vi "LS Durability Main (FPGA).vi"() -> ()   [LabVIEW 2013]
uses:
  <vilib>/rvi/Emulation/niFpgaSctlEmulationGetInTimedLoop.vi
  <vilib>/rvi/Emulation/niFpgaEmulationReportErrorSimple.vi
  <vilib>/rvi/Emulation/niFpgaGetClockAttributes.vi
  <vilib>/rvi/DataTransferAndStorage/Container/Common/niFpgaContainerExecOnDevCompGetState.vi
  <vilib>/rvi/FIFO/Fifo_Resource/nirvififoEmulationWriteFpgaImpl.vi
  <vilib>/rvi/DataTransferAndStorage/Container/Common/niFpgaContainerGetUniqueNameForEmu.vi
  <vilib>/rvi/interface/RandomDataEmulation/nirviRandomDataFPGAFIFO.vi
  <vilib>/rvi/interface/RandomDataEmulation/niFpgaRandomDataHandleErrors.vi
  <vilib>/rvi/eio/common/nirviEmuReportErrorAndStop.vi
  <vilib>/rvi/Emulation/niFpgaCriticalErrorInLSC.vi
  <vilib>/rvi/eio/common/nirviEmuTemplateMethod_errors.vi
  <vilib>/rvi/DataTransferAndStorage/Container/XNode/niFpgaContainer.xnode
  <vilib>/rvi/FIFO/Fifo_Resource/niFpgaFifoEmulationRefIn.vi
  <vilib>/eio/EIONode/EIONode.xnode
panel:
  out "FIFO microseconds":u32
  in  "V(T)/R(F)":bool=TRUE
  in  "Resistance In":fxp<+/-,28,17>[](array[numeric])=[0.0, 0.0, 0.0, 0.0, 0.0, 0.0, 0.0, 0.0, 0.0, 0.0, 0.0, 0.0]
  in  "Subtract Noise":bool
  out "Anomaly Array":fxp<+/-,29,18>[](array[numeric])
  in  "Enable2ndStepCheck":bool
  out "Anomaly Resamples":fxp<+/-,28,17>[](array[numeric])
  in  "Anomaly Threshold":fxp<+/-,28,17>=0.02978515625
  out "Bank2Active":bool
  out "Bank1Active":bool
  out "Bank2On":bool
  out "Bank1On":bool
  in  "Enable Readings":bool[](array[boolean])=[FALSE, FALSE, FALSE, FALSE, FALSE, FALSE, FALSE, FALSE, FALSE, FALSE, FALSE, FALSE]
  in  "Opens Resets":bool[](array[boolean])=[FALSE, FALSE, FALSE, FALSE, FALSE, FALSE, FALSE, FALSE, FALSE, FALSE, FALSE, FALSE]
  in  "Enable Opens":bool[](array[boolean])=[FALSE, FALSE, FALSE, FALSE, FALSE, FALSE, FALSE, FALSE, FALSE, FALSE, FALSE, FALSE]
  out "Opens Detected":u16[](array[numeric])
  out "Opens Loop Time (usec)":u32=1000
  in  "Bank2(Pulse/Const)":bool
  in  "Bank2Const(On/Off)":bool
  out "Anomalies (Last Cycle)":i32[](array[numeric])
  out "Cycle Starts":bool[](array[boolean])
  out "Anomalies (Total)":i32[](array[numeric])
  out "Anomalies/Cycle":i32[](array[numeric])
  in  "Normal Steps":u32=98
  out "Cycles":u32[](array[numeric])
  out "Anomaly Loop Time (usec)":u32=1000
  out "Steps":u32[](array[numeric])
  in  "Step Threshold":fxp<+/-,28,17>=0.02978515625
  in  "Enable Anomalies":bool[](array[boolean])=[FALSE, FALSE, FALSE, FALSE, FALSE, FALSE, FALSE, FALSE, FALSE, FALSE, FALSE, FALSE]
  in  "Anomaly Resets":bool[](array[boolean])=[FALSE, FALSE, FALSE, FALSE, FALSE, FALSE, FALSE, FALSE, FALSE, FALSE, FALSE, FALSE]
  in  "Bank1Const(On/Off)":bool
  in  "Bank1(Pulse/Const)":bool
  in  "PWM Period (Ticks)":u32=4000000
  in  "Duty (Ticks)":i32=2000000
  in  "Invert PWM?":bool=TRUE
  in  "Cycle Resets":bool[](array[boolean])=[FALSE, FALSE, FALSE, FALSE, FALSE, FALSE, FALSE, FALSE, FALSE, FALSE, FALSE, FALSE]
  in  "Points to Avg":i32=20
  in  "Enable Cycles":bool[](array[boolean])=[FALSE, FALSE, FALSE, FALSE, FALSE, FALSE, FALSE, FALSE, FALSE, FALSE, FALSE, FALSE]
  out "Total Cycles":u32[](array[numeric])
  in  "Cycle Threshold":fxp<+/-,28,17>=1.2001953125
  out "AI Avg Loop Time (usec)":u32=1000
  out "Analog Inputs":fxp<+/-,28,17>[](array[numeric])
  out "AI Loop Time (usec)":u32=70
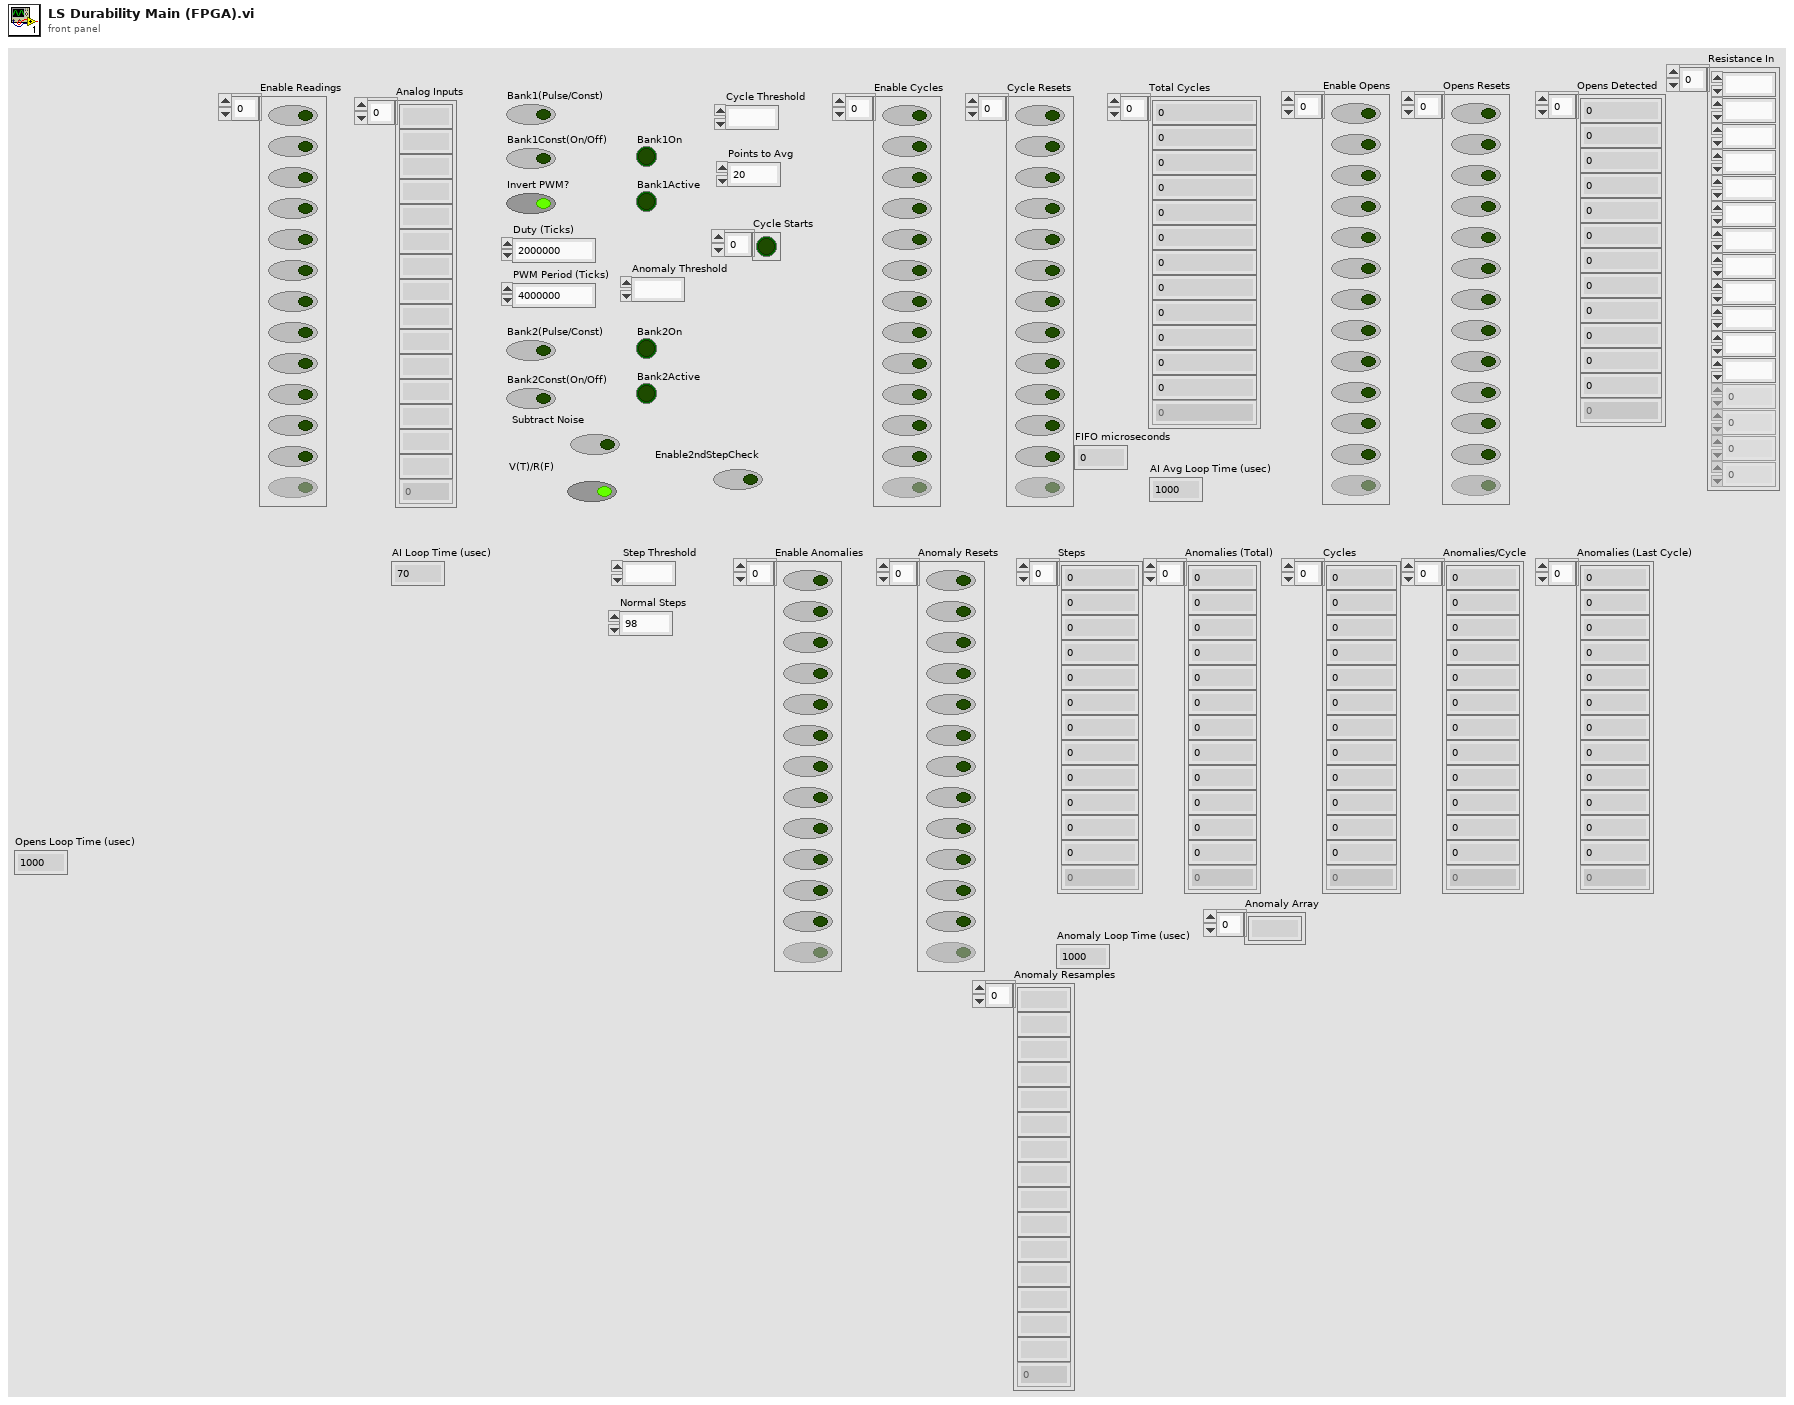
[diagram p1: front panel]
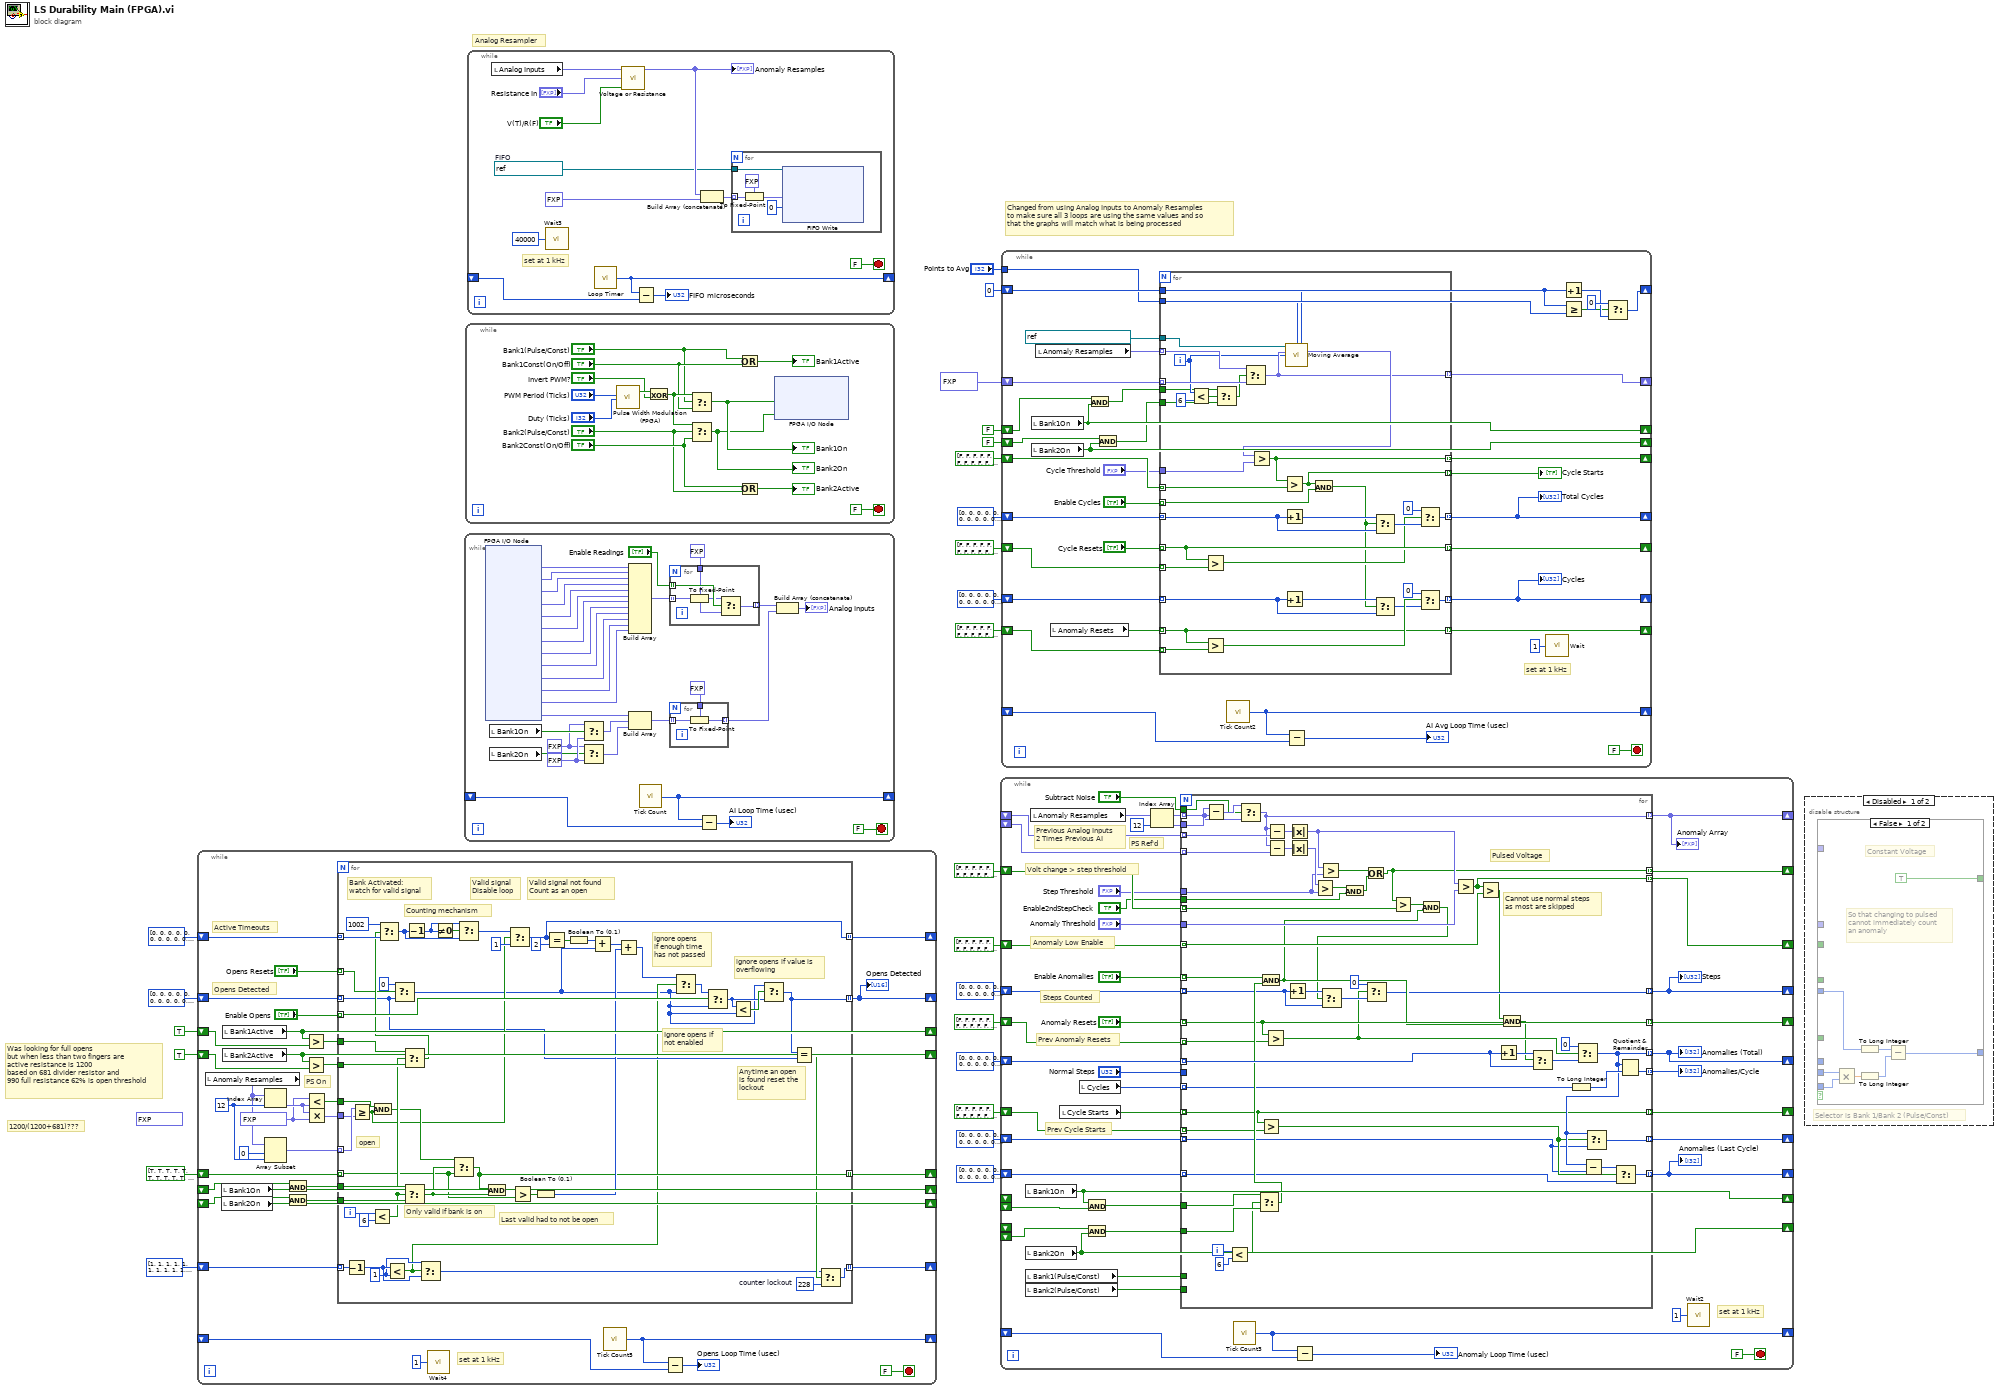
[diagram p0: block diagram]
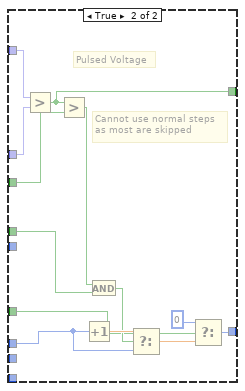
[diagram p2: hidden frame]
diagram:
  (unwired) fxp<+,8,0> 0.94921875
  # "Changed from using Analog Inputs to Anomaly Resamples\nto make sure all 3 loops are using the same values and so\nthat the graphs will match what is being processed"
  # "Analog Resampler"
  # "1200/(1200+681)???"
  # "Was looking for full opens\nbut when less than two fingers are\nactive resistance is 1200\nbased on 681 divider resistor and\n990 full resistance 62% is open threshold"
  n1 = while {
    shift-right: [w57] -> _
    shift-left: _ -> [w56]
    shift-right: [w28] -> _
    shift-left: u8[] [0, 0, 0, 0, 0, 0, 0, 0, 0, 0, 0, 0] -> [w52]
    shift-right: [w37] -> _
    shift-left: u16[] [0, 0, 0, 0, 0, 0, 0, 0, 0, 0, 0, 0] -> [w38]
    shift-right: [w44] -> _
    shift-left: bool[] [TRUE, TRUE, TRUE, TRUE, TRUE, TRUE, TRUE, TRUE, TRUE, TRUE, TRUE, TRUE] -> [w43]
    shift-right: [w42] -> _
    shift-left: TRUE ("Bank2Active") -> [w40]
    shift-right: [w41] -> _
    shift-left: TRUE ("Bank1Active") -> [w39]
    shift-right: [w31] -> _
    shift-left: _ -> [w29]
    shift-right: [w32] -> _
    shift-left: _ -> [w30]
    shift-right: [w26] -> _
    shift-left: u16[] [1, 1, 1, 1, 1, 1, 1, 1, 1, 1, 1, 1] -> [w27]
    stop <- FALSE stop-if-true
    w45 = fxp<+,8,0> 0.62109375
    w54 = 12 ("length")
    # "Opens Detected"
    # "Active Timeouts"
    # "PS On"
    # "set at 1 kHz"
    n2 = local read "Anomaly Resamples"() -> (w25:fxp<+/-,28,17>[])
    n3 = local read "Bank1On"() -> (w32:bool)
    n4 = local read "Bank2On"() -> (w31:bool)
    n5 = local read "Bank1Active"() -> (w41:bool)
    n6 = local read "Bank2Active"() -> (w42:bool)
    n7 = Index Array(array=w25, index=w54) -> (element=w46:fxp<+/-,28,17>)
    n8 = Array Subset(array=w25, index=0, length=w54) -> (w47:fxp<+/-,28,17>[])
    n9 = And(x=w30, y=w32) -> (x .and. y?=w34:bool)
    n10 = And(x=w29, y=w31) -> (x .and. y?=w33:bool)
    n11 = Greater?(x=w41, y=w39) -> (0:w51:bool)
    n12 = Greater?(x=w42, y=w40) -> (0:w50:bool)
    n13 = Less?(x=w45, y=w46) -> (x < y?=w49:bool)
    n14 = Multiply(x=w46, y=w45) -> (x*y=w48:fxp<+/-,36,17>)
    n15 = for {
      tunnel: w34 -> [w106]
      tunnel: w33 -> [w105]
      tunnel: w51 -> [w103]
      tunnel: w50 -> [w104]
      tunnel: w52 -> [w64] mode=indexing
      tunnel: w38 -> [w91] mode=indexing
      tunnel: "Opens Resets" -> [w75] mode=indexing
      tunnel: "Enable Opens" -> [w89] mode=indexing
      tunnel: [w65] -> w28 mode=indexing
      tunnel: w48 -> [w86]
      tunnel: w47 -> [w87] mode=indexing
      tunnel: w49 -> [w85]
      tunnel: [w76] -> w44 mode=indexing
      tunnel: w43 -> [w81] mode=indexing
      tunnel: [w79] -> w37 mode=indexing
      tunnel: w27 -> [w70] mode=indexing
      tunnel: [w66] -> w26 mode=indexing
      i -> [w108]
      w67 = u16 228  # counter lockout
      w71 = u16 1 ("y")
      # "Ignore opens if\nnot enabled"
      # "Ignore opens\nif enough time\nhas not passed"
      # "Anytime an open\nis found reset the\nlockout"
      # "ignore opens if value is\noverflowing"
      # "Last valid had to not be open"
      # "Only valid if bank is on"
      # "open"
      # "Valid signal not found\nCount as an open"
      # "Valid signal\nDisable loop"
      # "Counting mechanism"
      # "Bank Activated:\nwatch for valid signal"
      n16 = Decrement(x=w70) -> (x-1=w72:u16)
      n17 = Greater Or Equal?(x=w87, y=w86) -> (x >= y?=w78:bool)
      n18 = Less?(x=w108, y=6) -> (x < y?=w102:bool)
      n19 = And(x=w85, y=w78) -> (x .and. y?=w84:bool)
      n20 = Less?(x=w72, y=w71) -> (x < y?=w61:bool)
      n21 = Select(t=u16 0, s=w75, f=w64) -> (s? t:f=w60:u16)
      n22 = Select(t=w103, s=w102, f=w104) -> (s? t:f=w88:bool)
      n23 = Select(t=u16 1002, s=w88, f=w91) -> (s? t:f=w90:u16)
      n24 = Select(t=w106, s=w102, f=w105) -> (s? t:f=w83:bool)
      n25 = Decrement(x=w90) -> (x-1=w95:u16)
      n26 = Select(t=w71, s=w61, f=w72) -> (s? t:f=w68:u16)
      n27 = Not Equal To 0?(x=w95) -> (x != 0?=w94:bool)
      n28 = Select(t=w84, s=w83, f=w81) -> (s? t:f=w76:bool)
      n29 = Select(t=w95, s=w94, f=w90) -> (s? t:f=w96:u16)
      n30 = And(x=w76, y=w83) -> (x .and. y?=w77:bool)
      n31 = Select(t=w96, s=w78, f=u16 1) -> (s? t:f=w79:u16)
      n32 = Greater?(x=w77, y=w81) -> (0:w82:bool)
      n33 = Boolean To (0,1)(Boolean=w82) -> (0, 1=w80:i16)
      n34 = Equal?(x=w79, y=u16 2) -> (x = y?=w98:bool)
      n35 = Boolean To (0,1)(Boolean=w98) -> (0, 1=w99:i16)
      n36 = Add(x=w99, y=w60) -> (x+y=w100:u16)
      n37 = Add(x=w100, y=w80) -> (x+y=w62:u16)
      n38 = Select(t=w62, s=w61, f=w60) -> (s? t:f=w63:u16)
      n39 = Select(t=w63, s=w89, f=w60) -> (s? t:f=w73:u16)
      n40 = Less?(x=w73, y=w60) -> (x < y?=w74:bool)
      n41 = Select(t=w60, s=w74, f=w73) -> (s? t:f=w65:u16)
      n42 = Equal?(x=w65, y=w64) -> (x = y?=w69:bool)
      n43 = Select(t=w68, s=w69, f=w67) -> (s? t:f=w66:u16)
    }
    "Opens Detected" <- w28
    n44 = call "Wait4"("Count(mSec)"=u32 1) -> ()  [unwired: 1 out]
    n45 = call "Tick Count5"() -> ("Tick Count(uSec)"=w57:u32)
    n46 = Subtract(x=w57, y=w56) -> (x-y=→"Opens Loop Time (usec)":u32)
  }
  n47 = while {
    shift-right: [w138] -> _
    shift-left: _ -> [w137]
    stop <- FALSE stop-if-true
    w111 = fxp<+/-,24,5> 1.0 ("AI13")
    w114 = fxp<+/-,24,5> 0.0 ("AI13")
    n48 = xnode "FPGA I/O Node"() -> ("AI0"=w135:fxp<+/-,24,5>, "AI1"=w134:fxp<+/-,24,5>, "AI2"=w133:fxp<+/-,24,5>, "AI3"=w132:fxp<+/-,24,5>, "AI4"=w131:fxp<+/-,24,5>, "AI5"=w130:fxp<+/-,24,5>, "AI6"=w129:fxp<+/-,24,5>, "AI7"=w128:fxp<+/-,24,5>, "AI8"=w127:fxp<+/-,24,5>, "AI9"=w126:fxp<+/-,24,5>, "AI10"=w125:fxp<+/-,24,5>, "AI11"=w124:fxp<+/-,24,5>, "AI12"=w121:fxp<+/-,24,5>)  [unwired: 13 in, 13 out]
    n49 = local read "Bank1On"() -> (w113:bool)
    n50 = local read "Bank2On"() -> (w112:bool)
    n51 = Select(t=w111, s=w113, f=w114) -> (s? t:f=w110:fxp<+/-,24,5>)
    n52 = Select(t=w111, s=w112, f=w114) -> (s? t:f=w109:fxp<+/-,24,5>)
    n53 = Build Array(w135, w134, w133, w132, w131, w130, w129, w128, w127, w126, w125, w124) -> (w123:fxp<+/-,24,5>[])
    n54 = Build Array(w121, w110, w109) -> (w119:fxp<+/-,24,5>[])
    n55 = call "Tick Count"() -> ("Tick Count(uSec)"=w138:u32)
    n56 = for {
      tunnel: w123 -> [w147] mode=indexing
      tunnel: fxp<+/-,28,17> 0.0 ("AI0") -> [w144]
      tunnel: [w143] -> w117 mode=indexing
      tunnel: "Enable Readings" -> [w146] mode=indexing
      n57 = To Fixed-Point(fixed-point type=w144, number=w147) -> (fixed-point=w145:fxp<+/-,28,17>)
      n58 = Select(t=w145, s=w146, f=w144) -> (s? t:f=w143:fxp<+/-,28,17>)
    }
    n59 = for {
      tunnel: w119 -> [w142] mode=indexing
      tunnel: fxp<+/-,28,17> 0.0 ("AI0") -> [w141]
      tunnel: [w140] -> w118 mode=indexing
      n60 = To Fixed-Point(fixed-point type=w141, number=w142) -> (fixed-point=w140:fxp<+/-,28,17>)
    }
    n61 = Subtract(x=w138, y=w137) -> (x-y=→"AI Loop Time (usec)":u32)
    n62 = Build Array (concatenate)(w117, w118) -> (→"Analog Inputs":fxp<+/-,28,17>[])
  }
  n63 = while {
    stop <- FALSE stop-if-true
    n64 = call "Pulse Width Modulation (FPGA).vi"("PWM Period (Ticks)"="PWM Period (Ticks)", "PWM Duty Cycle (Ticks)"="Duty (Ticks)") -> ("PWM DO"=w158:bool)  [unwired: 14 in, 3 out]
    n65 = Exclusive Or(1:"Invert PWM?", 2:w158) -> (0:w156:bool)
    n66 = Select(t=w156, s="Bank1(Pulse/Const)", f="Bank1Const(On/Off)") -> (s? t:f=w155:bool)
    "Bank1On" <- w155
    n67 = Select(t=w156, s="Bank2(Pulse/Const)", f="Bank2Const(On/Off)") -> (s? t:f=w154:bool)
    "Bank2On" <- w154
    n68 = Or(x="Bank1(Pulse/Const)", y="Bank1Const(On/Off)") -> (x .or. y?=→"Bank1Active":bool)
    n69 = Or(x="Bank2Const(On/Off)", y="Bank2(Pulse/Const)") -> (x .or. y?=→"Bank2Active":bool)
    n70 = xnode "FPGA I/O Node"("RMC/DIO0"=w155, "RMC/DIO1"=w154) -> ()  [unwired: 3 in, 3 out]
  }
  n71 = while {
    shift-right: [w163] -> _
    shift-left: _ -> [w164]
    stop <- FALSE stop-if-true
    w165 = refnum<k21> "Analog Data"  # FIFO
    # "set at 1 kHz"
    n72 = local read "Analog Inputs"() -> (w169:fxp<+/-,28,17>[])
    n73 = call "Wait3"("Count(Ticks)"=u32 40000 ("Count(mSec)")) -> ()  [unwired: 1 out]
    n74 = call "Loop Timer"() -> ("Tick Count(uSec)"=w163:u32)  [unwired: 1 in]
    n75 = call "Voltage or Resistance.vi"("Data In"=w169, "Resistance In"="Resistance In", "V(T)/R(F)"="V(T)/R(F)") -> ("Data Out"=w168:fxp<+/-,28,17>[])  [unwired: 12 in]
    "Anomaly Resamples" <- w168
    n76 = Subtract(x=w163, y=w164) -> (x-y=→"FIFO microseconds":u32)
    n77 = Build Array (concatenate)(w168, fxp<+/-,28,17> -15.0 ("AI0")) -> (w172:fxp<+/-,28,17>[])
    n78 = for {
      tunnel: w165 -> [w178]
      tunnel: w172 -> [w177] mode=indexing
      n79 = To Fixed-Point(fixed-point type=fxp<+/-,18,11> 0.0 ("AI0"), number=w177) -> (fixed-point=w176:fxp<+/-,18,11>)
      n80 = xnode "FIFO Write"("Element"=w176, "Timeout"=0, "FIFO In"=w178) -> ()  [unwired: 2 out]
    }
  }
  n81 = while {
    shift-right: [w220] -> _
    shift-left: _ -> [w219]
    shift-right: [w212] -> _
    shift-left: bool[] [FALSE, FALSE, FALSE, FALSE, FALSE, FALSE, FALSE, FALSE, FALSE, FALSE, FALSE, FALSE] -> [w211]
    shift-right: [w209] -> _
    shift-left: u32[] [0, 0, 0, 0, 0, 0, 0, 0, 0, 0, 0, 0] -> [w208]
    shift-right: [w207] -> _
    shift-left: bool[] [FALSE, FALSE, FALSE, FALSE, FALSE, FALSE, FALSE, FALSE, FALSE, FALSE, FALSE, FALSE] -> [w204]
    shift-right: [w214] -> _
    shift-left: _ -> [w213]
    shift-right: [w201] -> _
    shift-left: bool[] [FALSE, FALSE, FALSE, FALSE, FALSE, FALSE, FALSE, FALSE, FALSE, FALSE, FALSE, FALSE] -> [w200]
    shift-right: [w199] -> _
    shift-left: i32[] [0, 0, 0, 0, 0, 0, 0, 0, 0, 0, 0, 0] -> [w197]
    shift-right: [w198] -> _
    shift-left: i32[] [0, 0, 0, 0, 0, 0, 0, 0, 0, 0, 0, 0] -> [w196]
    shift-right: [w188] -> _
    shift-left: _ -> [_]
    shift-right: [w215] -> _
    shift-left: _ -> [_]
    shift-right: [w193] -> _
    shift-left: i32[] [0, 0, 0, 0, 0, 0, 0, 0, 0, 0, 0, 0] -> [w192]
    shift-right: [w189] -> _
    shift-left: bool[] [FALSE, FALSE, FALSE, FALSE, FALSE, FALSE, FALSE, FALSE, FALSE, FALSE, FALSE, FALSE] -> [w190]
    shift-left: _ -> [w186]
    shift-left: _ -> [w187]
    shift-left: _ -> [w184]
    stop <- FALSE stop-if-true
    # "PS Ref'd"
    # "Anomaly Low Enable"
    # "Prev Cycle Starts"
    # "Prev Anomaly Resets"
    # "Steps Counted"
    # "Volt change > step threshold"
    # "Previous Analog Inputs\n2 Times Previous AI"
    # "set at 1 kHz"
    n82 = local read "Bank1On"() -> (w188:bool)
    n83 = local read "Bank2On"() -> (w215:bool)
    n84 = local read "Bank1(Pulse/Const)"() -> (w195:bool)
    n85 = local read "Bank2(Pulse/Const)"() -> (w194:bool)
    n86 = local read "Anomaly Resamples"() -> (w182:fxp<+/-,28,17>[])
    n87 = local read "Cycle Starts"() -> (w202:bool[])
    n88 = local read "Cycles"() -> (w203:u32[])
    n89 = And(x=w188, y=w187) -> (x .and. y?=w217:bool)
    n90 = And(x=w186, y=w215) -> (x .and. y?=w216:bool)
    n91 = Index Array(array=w182, index=12) -> (element=w181:fxp<+/-,28,17>)
    n92 = for {
      tunnel: w182 -> [w225] mode=indexing
      tunnel: [w232] -> w212 mode=indexing
      tunnel: w211 -> [w253] mode=indexing
      tunnel: w208 -> [w246] mode=indexing
      tunnel: [w245] -> w209 mode=indexing
      tunnel: "Step Threshold" -> [w234]
      tunnel: "Enable Anomalies" -> [w272] mode=indexing
      tunnel: "Anomaly Resets" -> [w255] mode=indexing
      tunnel: [w255] -> w207 mode=indexing
      tunnel: w204 -> [w256] mode=indexing
      tunnel: [w226] -> w214 mode=indexing
      tunnel: w213 -> [w273] mode=indexing
      tunnel: "Normal Steps" -> [_]
      tunnel: w203 -> [w263] mode=indexing
      tunnel: [w262] -> w205 mode=indexing
      tunnel: [w264] -> w193 mode=indexing
      tunnel: w202 -> [w258] mode=indexing
      tunnel: [w258] -> w201 mode=indexing
      tunnel: w200 -> [w259] mode=indexing
      tunnel: [w261] -> w199 mode=indexing
      tunnel: w197 -> [w244] mode=indexing
      tunnel: [w260] -> w198 mode=indexing
      tunnel: w196 -> [w243] mode=indexing
      tunnel: w217 -> [w280]
      tunnel: w216 -> [w279]
      tunnel: w195 -> [_]
      tunnel: w194 -> [_]
      tunnel: w192 -> [w275] mode=indexing
      tunnel: "Anomaly Threshold" -> [w269]
      tunnel: w190 -> [w268] mode=indexing
      tunnel: [w267] -> w189 mode=indexing
      tunnel: w184 -> [w236] mode=indexing
      tunnel: "Enable2ndStepCheck" -> [w229]
      tunnel: w181 -> [w228]
      tunnel: "Subtract Noise" -> [w224]
      i -> [w278]
      # "Cannot use normal steps\nas most are skipped"
      # "Pulsed Voltage"
      n93 = Subtract(x=w228, y=w225) -> (x-y=w227:fxp<+/-,29,18>)
      n94 = Less?(x=w278, y=6) -> (x < y?=w276:bool)
      n95 = Select(t=w227, s=w224, f=w225) -> (s? t:f=w226:fxp<+/-,29,18>)
      n96 = Select(t=w280, s=w276, f=w279) -> (s? t:f=w271:bool)
      n97 = And(x=w272, y=w271) -> (x .and. y?=w252:bool)
      n98 = Greater?(x=w258, y=w259) -> (0:w257:bool)
      n99 = Greater?(x=w255, y=w256) -> (0:w248:bool)
      n100 = Subtract(x=w226, y=w273) -> (x-y=w274:fxp<+/-,30,19>)
      n101 = Subtract(x=w226, y=w236) -> (x-y=w237:fxp<+/-,30,19>)
      n102 = Increment(x=w246) -> (x+1=w249:u32)
      n103 = Absolute Value(x=w274) -> (abs(x)=w270:fxp<+,29,18>)
      n104 = Absolute Value(x=w237) -> (abs(x)=w235:fxp<+,29,18>)
      n105 = Greater?(x=w235, y=w234) -> (0:w231:bool)
      n106 = Greater?(x=w270, y=w234) -> (0:w233:bool)
      n107 = And(x=w231, y=w229) -> (x .and. y?=w230:bool)
      n108 = Or(x=w233, y=w230) -> (x .or. y?=w232:bool)
      n109 = Greater?(x=w232, y=w253) -> (0:w254:bool)
      n110 = And(x=w254, y=w252) -> (x .and. y?=w247:bool)
      n111 = Select(t=w249, s=w247, f=w246) -> (s? t:f=w250:u32)
      n112 = Select(t=u32 0, s=w248, f=w250) -> (s? t:f=w245:u32)
      n113 = Greater?(x=w270, y=w269) -> (0:w267:bool)
      n114 = Greater?(x=w267, y=w268) -> (0:w238:bool)
      n115 = Increment(x=w275) -> (x+1=w240:i32)
      n116 = And(x=w238, y=w252) -> (x .and. y?=w239:bool)
      n117 = Select(t=w240, s=w239, f=w275) -> (s? t:f=w241:i32)
      n118 = To Long Integer(number=w263) -> (32bit integer=w265:i32)
      n119 = Select(t=0, s=w248, f=w241) -> (s? t:f=w264:i32)
      n120 = Subtract(x=w264, y=w244) -> (x-y=w266:i32)
      n121 = Select(t=w264, s=w257, f=w244) -> (s? t:f=w261:i32)
      n122 = Select(t=w266, s=w257, f=w243) -> (s? t:f=w260:i32)
      n123 = Quotient & Remainder(x=w264, y=w265) -> (floor(x/y)=w262:i32)  [unwired: 1 out]
    }
    "Steps" <- w209
    "Anomalies/Cycle" <- w205
    "Anomalies (Total)" <- w193
    "Anomalies (Last Cycle)" <- w198
    "Anomaly Array" <- w214
    n124 = call "Tick Count3"() -> ("Tick Count(uSec)"=w220:u32)
    n125 = Subtract(x=w220, y=w219) -> (x-y=→"Anomaly Loop Time (usec)":u32)
    n126 = call "Wait2"("Count(mSec)"=u32 1) -> ()  [unwired: 1 out]
  }
  n127 = while {
    shift-right: [w310] -> _
    shift-left: 0 ("Moving Point Index") -> [w311]
    shift-right: [w307] -> _
    shift-left: _ -> [w306]
    shift-right: [w305] -> _
    shift-left: bool[] [FALSE, FALSE, FALSE, FALSE, FALSE, FALSE, FALSE, FALSE, FALSE, FALSE, FALSE, FALSE] -> [w304]
    shift-right: [w302] -> _
    shift-left: u32[] [0, 0, 0, 0, 0, 0, 0, 0, 0, 0, 0, 0] -> [w303]
    tunnel: "Points to Avg" -> [w299]
    shift-right: [w297] -> _
    shift-left: bool[] [FALSE, FALSE, FALSE, FALSE, FALSE, FALSE, FALSE, FALSE, FALSE, FALSE, FALSE, FALSE] -> [w296]
    shift-right: [w291] -> _
    shift-left: u32[] [0, 0, 0, 0, 0, 0, 0, 0, 0, 0, 0, 0] -> [w293]
    shift-right: [w294] -> _
    shift-left: bool[] [FALSE, FALSE, FALSE, FALSE, FALSE, FALSE, FALSE, FALSE, FALSE, FALSE, FALSE, FALSE] -> [w295]
    shift-right: [w287] -> _
    shift-left: FALSE -> [w285]
    shift-right: [w283] -> _
    shift-left: FALSE -> [w284]
    shift-right: [w288] -> _
    shift-left: fxp<+/-,28,17>[] [0.0, 0.0, 0.0, 0.0, 0.0, 0.0, 0.0, 0.0, 0.0, 0.0, 0.0, 0.0] ("Analog Inputs") -> [w289]
    stop <- FALSE stop-if-true
    # "set at 1 kHz"
    n128 = local read "Bank1On"() -> (w287:bool)
    n129 = local read "Bank2On"() -> (w283:bool)
    n130 = local read "Anomaly Resamples"() -> (w281:fxp<+/-,28,17>[])
    n131 = local read "Anomaly Resets"() -> (w292:bool[])
    n132 = And(x=w285, y=w287) -> (x .and. y?=w286:bool)
    n133 = And(x=w284, y=w283) -> (x .and. y?=w282:bool)
    n134 = for {
      tunnel: w311 -> [w349]
      tunnel: w299 -> [w350]
      tunnel: w281 -> [w325] mode=indexing
      tunnel: refnum<k21> "Running Avg Memory" ("Memory") -> [w351]
      tunnel: [w348] -> w305 mode=indexing
      tunnel: w304 -> [w347] mode=indexing
      tunnel: w303 -> [w345] mode=indexing
      tunnel: [w337] -> w302 mode=indexing
      tunnel: "Cycle Threshold" -> [w344]
      tunnel: "Enable Cycles" -> [w343] mode=indexing
      tunnel: "Cycle Resets" -> [w342] mode=indexing
      tunnel: [w342] -> w297 mode=indexing
      tunnel: w296 -> [w341] mode=indexing
      tunnel: w293 -> [w330] mode=indexing
      tunnel: [w336] -> w291 mode=indexing
      tunnel: w292 -> [w331] mode=indexing
      tunnel: [w331] -> w294 mode=indexing
      tunnel: w295 -> [w332] mode=indexing
      tunnel: [w328] -> w290 mode=indexing
      tunnel: w289 -> [w326] mode=indexing
      tunnel: [w324] -> w288 mode=indexing
      tunnel: w286 -> [w319]
      tunnel: w282 -> [w318]
      i -> [w321]
      n135 = Less?(x=w321, y=6) -> (x < y?=w322:bool)
      n136 = Greater?(x=w342, y=w341) -> (0:w339:bool)
      n137 = Greater?(x=w331, y=w332) -> (0:w334:bool)
      n138 = Select(t=w319, s=w322, f=w318) -> (s? t:f=w320:bool)
      n139 = Select(t=w325, s=w320, f=w326) -> (s? t:f=w324:fxp<+/-,28,17>)
      n140 = Increment(x=w345) -> (x+1=w346:u32)
      n141 = Increment(x=w330) -> (x+1=w329:u32)
      n142 = call "Moving Average.vi"("Memory In"=w351, "N (# of Ave Pts 127 max)"=w350, "Moving Point Index"=w349, "Data IN"=w324, "Channel#"=w321) -> ("Averaged Data"=w327:fxp<+/-,28,17>)  [unwired: 10 in]
      n143 = Greater?(x=w327, y=w344) -> (0:w348:bool)
      n144 = Greater?(x=w348, y=w347) -> (0:w328:bool)
      n145 = And(x=w328, y=w343) -> (x .and. y?=w317:bool)
      n146 = Select(t=w346, s=w317, f=w345) -> (s? t:f=w340:u32)
      n147 = Select(t=w329, s=w317, f=w330) -> (s? t:f=w333:u32)
      n148 = Select(t=u32 0, s=w339, f=w340) -> (s? t:f=w337:u32)
      n149 = Select(t=u32 0, s=w334, f=w333) -> (s? t:f=w336:u32)
    }
    "Total Cycles" <- w302
    "Cycles" <- w291
    "Cycle Starts" <- w290
    n150 = call "Tick Count2"() -> ("Tick Count(uSec)"=w307:u32)
    n151 = Subtract(x=w307, y=w306) -> (x-y=→"AI Avg Loop Time (usec)":u32)
    n152 = call "Wait"("Count(mSec)"=u32 1) -> ()  [unwired: 1 out]
    n153 = Increment(x=w311) -> (x+1=w313:i32)
    n154 = Greater Or Equal?(x=w311, y=w299) -> (x >= y?=w312:bool)
    n155 = Select(t=0, s=w312, f=w313) -> (s? t:f=w310:i32)
  }
  n156 = disable-structure shown="Disabled" {
    frame Disabled {
      # "Selector is Bank 1/Bank 2 (Pulse/Const)"
      n157 = case shown="False" {
        selector: _ -> [_ _]
        tunnel: _ -> [w359 _]
        tunnel: _ -> [w355 _]
        tunnel: [w354 w368] -> _
        tunnel: _ -> [w352 _]
        tunnel: _ -> [_ w369]
        tunnel: _ -> [_ w365]
        tunnel: _ -> [_ w366]
        tunnel: _ -> [_ w364]
        tunnel: _ -> [_ w363]
        tunnel: [TRUE w362] -> _
        tunnel: _ -> [_ w360]
        frame False {
          # "So that changing to pulsed\ncannot immediately count\nan anomaly"
          # "Constant Voltage"
          n158 = Multiply(x=w359, y=w355) -> (x*y=w358:dbl)
          n159 = To Long Integer(number=w352) -> (32bit integer=w357:i32)
          n160 = To Long Integer(number=w358) -> (32bit integer=w356:i32)
          n161 = Subtract(x=w357, y=w356) -> (x-y=w354:i32)
        }
        frame True {
          # "Cannot use normal steps\nas most are skipped"
          # "Pulsed Voltage"
          n162 = Greater?(x=w365, y=w364) -> (0:w362:bool)
          n163 = Greater?(x=w362, y=w363) -> (0:w361:bool)
          n164 = Increment(x=w369) -> (x+1=w370:dbl)
          n165 = And(x=w361, y=w366) -> (x .and. y?=w367:bool)
          n166 = Select(t=w370, s=w367, f=w369) -> (s? t:f=w371:dbl)
          n167 = Select(t=0, s=w360, f=w371) -> (s? t:f=w368:i32)
        }
      }
    }
    frame Enabled {
    }
  }
